vi "Configure Arm Source.vi"(7 "Detection (Rise)":i32(ring) items=["Rise", "Fall", "High", "Low"], 8 "error in (no error)":errorcluster {"code" format="%.0x"}, 9 "Enabled (Off)":bool, 10 "SourceName":string="LXI0" caption="SourceName (LXI0)", 11 "instrument handle":refnum<k15>) -> (0 "error out":errorcluster {"code" format="%.0x"}, 3 "instrument handle out":refnum<k15>)   [LabVIEW 2009, in "Keysight XSAn.lvlib"]
doc: "This VI configures the most commonly configured properties of the arm source sub-system.\n\nSupported Models: N9000A, N9000B, N9010A, N9010B, N9020A, N9020B, N9030A, N9030B, N9038A, SPN9003A, SPN9026A"
uses:
  <instrlib>/Keysight XSAn/Keysight XSAn.lvlib
  AgXSAn.dll
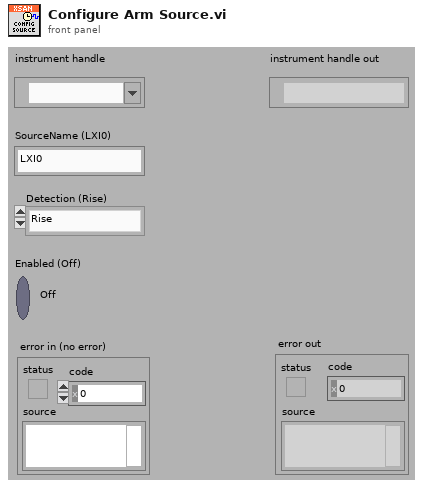
[diagram p1: front panel]
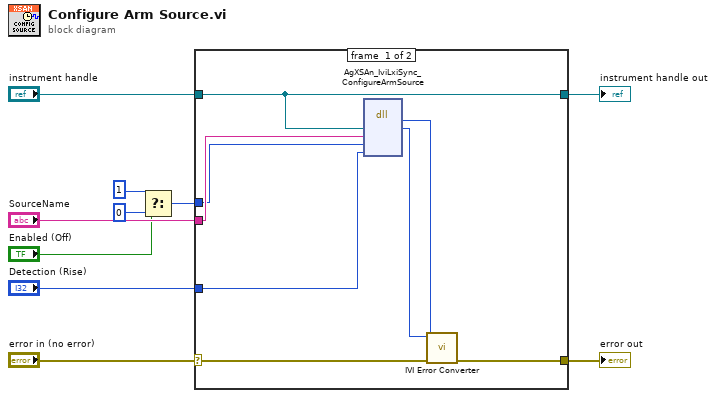
[diagram p0: block diagram]
diagram:
  n1 = Select(t=u16 1, s="Enabled (Off)", f=u16 0) -> (s? t:f=w3:u16)
  n2 = case shown="No Error" "error in (no error)" {
    selector: "error in (no error)" -> [w16 w20]
    tunnel: [w15 w20] -> w10
    tunnel: "instrument handle" -> [w11 w19]
    tunnel: "SourceName" -> [w14 _]
    tunnel: w3 -> [w13 _]
    tunnel: "Detection (Rise)" -> [w12 _]
    tunnel: [w11 w19] -> w1
    frame #0 {
      n3 = dll-call lib="AgXSAn**.dll" fn="AgXSAn_IviLxiSync_ConfigureArmSource"("Vi"=w11, "SourceName"=w14, "Enabled"=w13, "Detection"=w12) -> (w17:i32, "Vi"=w18:u32)  [unwired: 6 in, 2 out]
      n4 = call <instrlib>:"IVI Error Converter.vi"("error in (no error)"=w16, "IVI error code (0)"=w17, "instrument handle"=w18) -> ("error out"=w15:errorcluster)  [unwired: 7 in, 1 out]
    }
    frame #1 {
    }
  }
  "error out" <- w10
  "instrument handle out" <- w1
